vi "fibanoci and sum of n numbers.vi"() -> ()   [LabVIEW 2020]
panel:
  out "Numeric":dbl
  out "Array":dbl[](array[numeric])
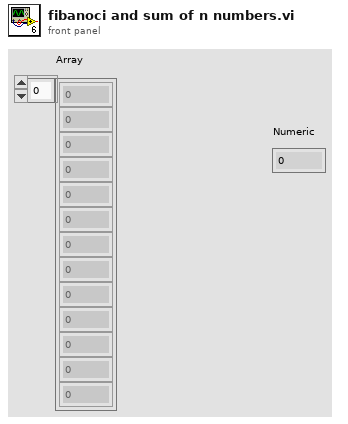
[diagram p1: front panel]
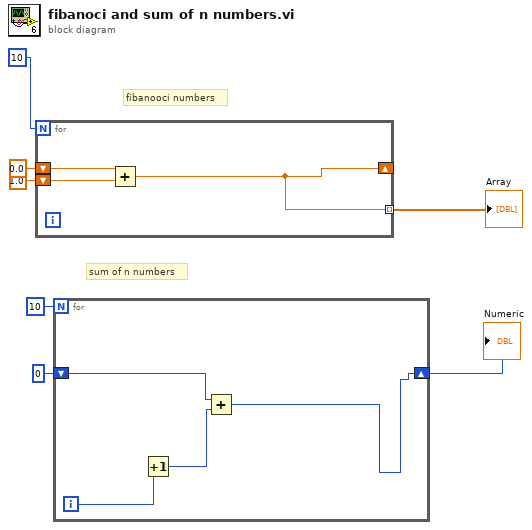
[diagram p0: block diagram]
diagram:
  # "fibanooci numbers"
  # "sum of n numbers"
  n1 = for {
    N: 10 -> [_]
    shift-right: [w8] -> _
    shift-left: 0.0 -> [w10]
    shift-left: 1.0 -> [w9]
    tunnel: [w8] -> w4 mode=indexing
    n2 = Add(x=w10, y=w9) -> (x+y=w8:dbl)
  }
  "Array" <- w4
  n3 = for {
    N: 10 -> [_]
    shift-right: [w11] -> w2
    shift-left: 0 -> [w13]
    i -> [w14]
    n4 = Increment(x=w14) -> (x+1=w12:i32)
    n5 = Add(x=w13, y=w12) -> (x+y=w11:i32)
  }
  "Numeric" <- w2
